vi "Make All Clumps.vi"(8 "Input.Input Registers":T7[](array[typedef]) {"Mapping"."VS Reference" format="%.0x"}, 9 "Output.Holding Registers":T7[](array[typedef]) {"Mapping"."VS Reference" format="%.0x"}, 10 "Input.Discrete Inputs":T7[](array[typedef]) {"Mapping"."VS Reference" format="%.0x"}, 11 "Output.Coils":T7[](array[typedef]) {"Mapping"."VS Reference" format="%.0x"}) -> (3 "Clumps":T1[](array[typedef]) {"Mappings"."VS Reference" format="%.0x"})   [LabVIEW 2021]
uses:
  <vilib>/NI VeriStand/Custom Device API/Custom Device Channel Type.ctl
  <vilib>/NI VeriStand/Custom Device API/Custom Device API.lvlib
  System Explorer/SubVIs/Modbus Type.ctl
  Shared/Modbus Master Shared.lvlib
  Shared/Controls/Data Model/DataType.ctl
  Shared/Controls/Data Model/Mapping.ctl
  Shared/Controls/Data Model/Channel.ctl
  Form Clump.ctl
  <vilib>/NI VeriStand/Custom Device API/Custom Device Item Ref.ctl
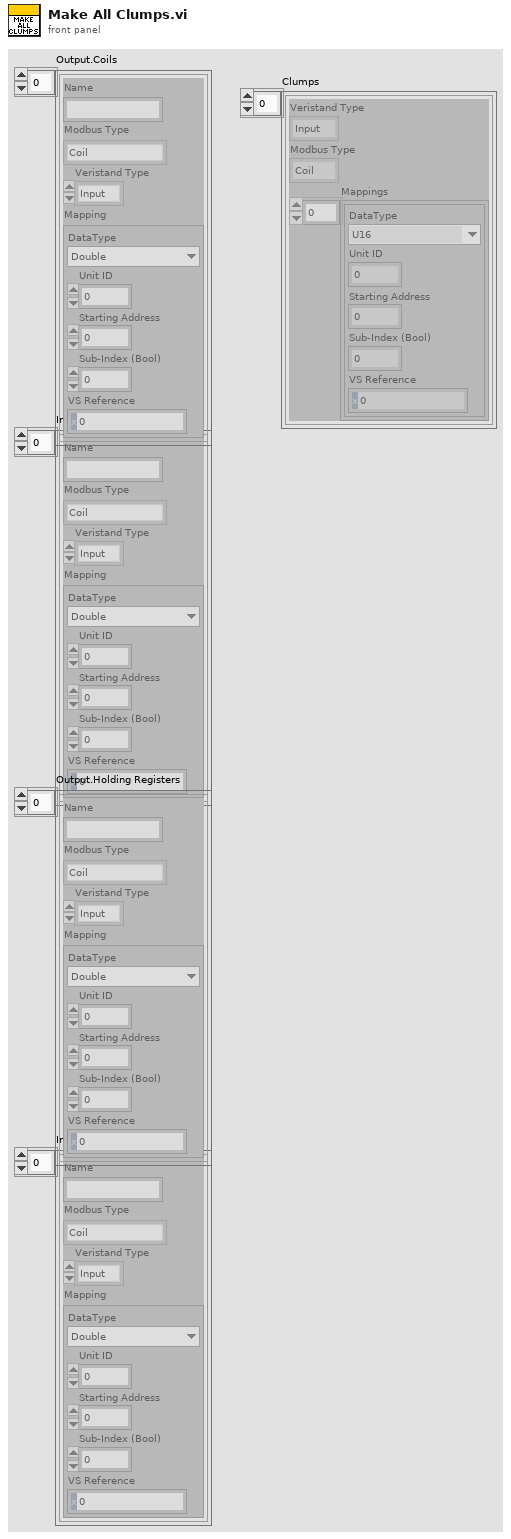
[diagram p1: front panel]
types:
  T1 = typedef "Modbus Master Shared.lvlib/Form Clump.ctl" = cluster{"Veristand Type":T2, "Modbus Type":T3, "Mappings":T4[]}
  T2 = typedef "Custom Device API.lvlib/Custom Device Channel Type.ctl" = enum16{"Input", "Output"}
  T3 = typedef "Modbus Master Shared.lvlib/Modbus Type.ctl" = enum16{"Coil", "Discrete Input", "Holding Register", "Input Register"}
  T4 = typedef "Modbus Master Shared.lvlib/Mapping.ctl" = cluster{"DataType":T5, "Unit ID":u8, "Starting Address":u16, "Sub-Index (Bool)":u16, "VS Reference":T6}
  T5 = typedef "Modbus Master Shared.lvlib/DataType.ctl" = enum16{"Double", "Single", "I64", "I32", "I16", "I8", "U64", "U32", "U16", "U8", "Boolean"}
  T6 = typedef "Custom Device API.lvlib/Custom Device Item Ref.ctl" = u64
  T7 = typedef "Modbus Master Shared.lvlib/Channel.ctl" = cluster{"Name":string, "Modbus Type":T3, "Veristand Type":T2, "Mapping":T4}
  T8 = typedef "Modbus Master Shared.lvlib/Form Clump.ctl" = cluster{"Veristand Type":T2, "Modbus Type":T3, "Mappings":T9[]}
  T9 = typedef "Modbus Master Shared.lvlib/Mapping.ctl" = cluster{"DataType":T5, "Starting Address":u16, "Sub-Index (Bool)":u16, "Reference Index":u16}
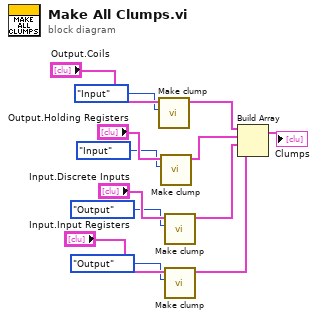
[diagram p0: block diagram]
diagram:
  n1 = call "Make clump.vi"("Veristand Type"=Custom_Device_Channel_Type."Input", "Channels"="Output.Coils") -> ("Cluster out"=w9:T8)  [unwired: 9 in]
  n2 = call "Make clump.vi"("Veristand Type"=Custom_Device_Channel_Type."Input", "Channels"="Output.Holding Registers") -> ("Cluster out"=w10:T8)  [unwired: 9 in]
  n3 = call "Make clump.vi"("Veristand Type"=Custom_Device_Channel_Type."Output", "Channels"="Input.Discrete Inputs") -> ("Cluster out"=w11:T8)  [unwired: 9 in]
  n4 = call "Make clump.vi"("Veristand Type"=Custom_Device_Channel_Type."Output", "Channels"="Input.Input Registers") -> ("Cluster out"=w12:T8)  [unwired: 9 in]
  n5 = Build Array(w9, w10, w11, w12) -> (→"Clumps":T8[])
